vi "testLoadLogFile.vi"() -> ()   [LabVIEW 2018]
uses:
  Read and Save Files/RW_Protocols.lvlib
panel:
  out "error out":errorcluster
  in  "sequence list":i32[](listbox)
  out "all values":dbl[][](array[numeric])
  out "Phase array unit":dbl[](array[numeric])
  out "sequence cluster":T1
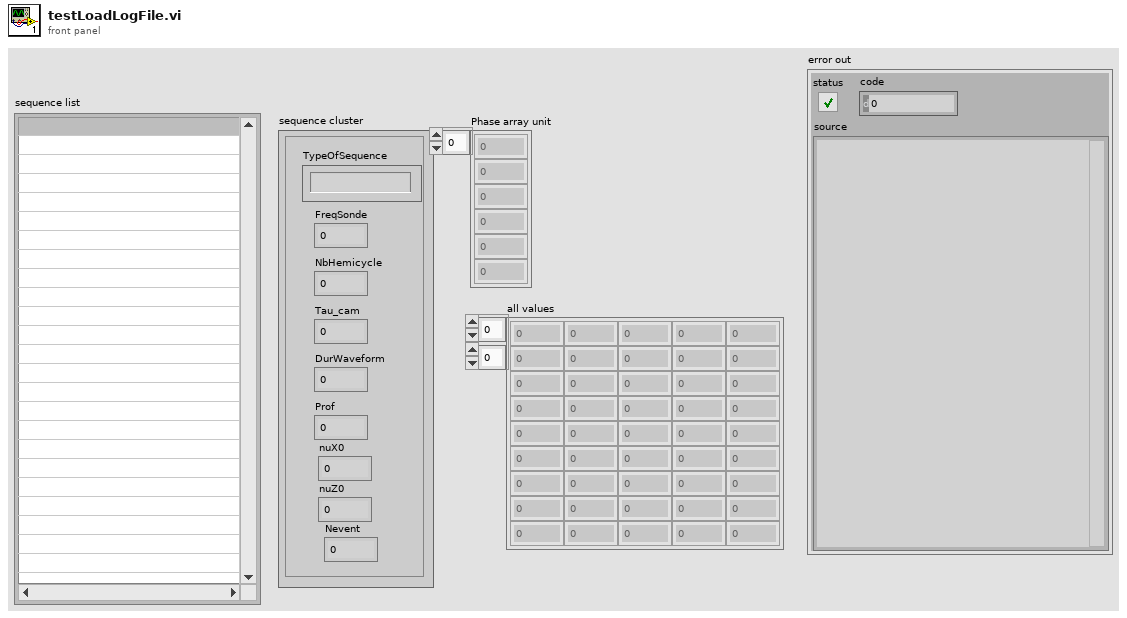
[diagram p1: front panel]
types:
  T1 = cluster{"TypeOfSequence":string, "FreqSonde":dbl, "NbHemicycle":dbl, "Tau_cam":dbl, "DurWaveform":dbl, "Prof":dbl, "Nevent":i32, "nuX0":dbl, "nuZ0":dbl}
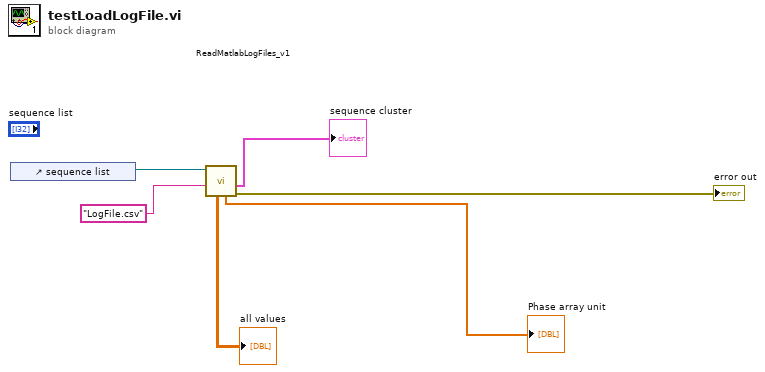
[diagram p0: block diagram]
diagram:
  n1 = control-ref of="sequence list"() -> (w5:refnum<vi>)
  n2 = call "ReadMatlabLogFiles_v1.vi"("FileName"="LogFile.csv", "sequence list REF"=w5) -> ("error out"=→"error out":errorcluster, "sequence cluster"=→"sequence cluster":T1, "Phase array unit"=→"Phase array unit":dbl[], "all values"=→"all values":dbl[][])  [unwired: 4 in, 2 out]
